vi "SetupEQE_ActiveX.vi"(6 "Skip?":bool, 8 "error in (no error)":errorcluster) -> (0 "error out":errorcluster)   [LabVIEW 2011]
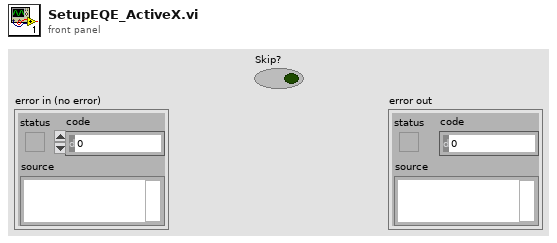
[diagram p1: front panel]
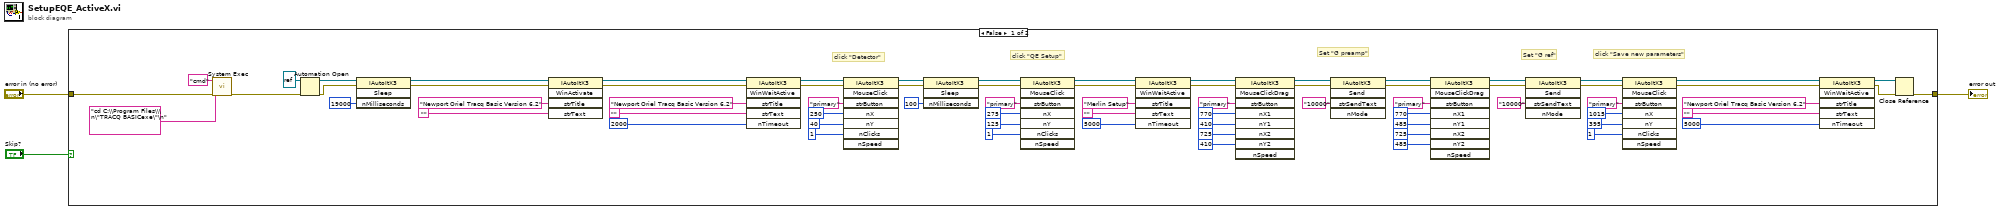
[diagram p0: block diagram]
diagram:
  n1 = case shown="False" "Skip?" {
    tunnel: "error in (no error)" -> [w6 w75]
    tunnel: [w72 w75] -> w2
    frame False {
      # "click \"Save new parameters\""
      # "Set \"G ref\""
      # "Set \"G preamp\""
      # "click \"QE Setup\""
      # "click \"Detector\""
      n2 = call <vilib>:"System Exec.vi"("error in (no error)"=w6, "standard input"="cd C:\\Program Files\\\n\"TRACQ BASICexe\"\n", "command line"="cmd") -> ("error out"=w5:errorcluster)  [unwired: 5 in, 3 out]
      n3 = Automation Open(error in (no error)=w5, Automation Refnum=refnum<k7> refnum ("AutoItX3Lib.IAutoItX3")) -> (Automation Refnum=w9:refnum<k7>, error out=w8:errorcluster)  [unwired: 2 in]
      n4 = invoke class="IAutoItX3" method="Sleep"(reference=w9, error in=w8, "nMilliseconds"=19000) -> (reference out=w70:refnum<k7>, error out=w71:errorcluster)  [unwired: 1 in, 2 out]
      n5 = invoke class="IAutoItX3" method="WinActivate"(reference=w70, error in=w71, "strTitle"="Newport Oriel Tracq Basic Version 6.2", "strText"="") -> (reference out=w69:refnum<k7>, error out=w62:errorcluster)  [unwired: 1 in, 3 out]
      n6 = invoke class="IAutoItX3" method="WinWaitActive"(reference=w69, error in=w62, "strTitle"="Newport Oriel Tracq Basic Version 6.2", "strText"="", "nTimeout"=2000) -> (reference out=w63:refnum<k7>, error out=w61:errorcluster)  [unwired: 1 in, 4 out]
      n7 = invoke class="IAutoItX3" method="MouseClick"(reference=w63, error in=w61, "strButton"="primary", "nX"=250, "nY"=40, "nClicks"=1) -> (reference out=w55:refnum<k7>, error out=w54:errorcluster)  [unwired: 2 in, 6 out]
      n8 = invoke class="IAutoItX3" method="Sleep"(reference=w55, error in=w54, "nMilliseconds"=100) -> (reference out=w49:refnum<k7>, error out=w48:errorcluster)  [unwired: 1 in, 2 out]
      n9 = invoke class="IAutoItX3" method="MouseClick"(reference=w49, error in=w48, "strButton"="primary", "nX"=275, "nY"=125, "nClicks"=1) -> (reference out=w44:refnum<k7>, error out=w43:errorcluster)  [unwired: 2 in, 6 out]
      n10 = invoke class="IAutoItX3" method="WinWaitActive"(reference=w44, error in=w43, "strTitle"="Merlin Setup", "strText"="", "nTimeout"=5000) -> (reference out=w42:refnum<k7>, error out=w41:errorcluster)  [unwired: 1 in, 4 out]
      n11 = invoke class="IAutoItX3" method="MouseClickDrag"(reference=w42, error in=w41, "strButton"="primary", "nX1"=770 ("nX"), "nY1"=410 ("nY"), "nX2"=725 ("nClicks"), "nY2"=410 ("nClicks")) -> (reference out=w35:refnum<k7>, error out=w34:errorcluster)  [unwired: 2 in, 7 out]
      n12 = invoke class="IAutoItX3" method="Send"(reference=w35, error in=w34, "strSendText"="10000") -> (reference out=w24:refnum<k7>, error out=w23:errorcluster)  [unwired: 2 in, 3 out]
      n13 = invoke class="IAutoItX3" method="MouseClickDrag"(reference=w24, error in=w23, "strButton"="primary", "nX1"=770 ("nX"), "nY1"=485 ("nY"), "nX2"=725 ("nClicks"), "nY2"=485 ("nClicks")) -> (reference out=w27:refnum<k7>, error out=w26:errorcluster)  [unwired: 2 in, 7 out]
      n14 = invoke class="IAutoItX3" method="Send"(reference=w27, error in=w26, "strSendText"="10000") -> (reference out=w18:refnum<k7>, error out=w17:errorcluster)  [unwired: 2 in, 3 out]
      n15 = invoke class="IAutoItX3" method="MouseClick"(reference=w18, error in=w17, "strButton"="primary", "nX"=1015, "nY"=395, "nClicks"=1) -> (reference out=w13:refnum<k7>, error out=w12:errorcluster)  [unwired: 2 in, 6 out]
      n16 = invoke class="IAutoItX3" method="WinWaitActive"(reference=w13, error in=w12, "strTitle"="Newport Oriel Tracq Basic Version 6.2", "strText"="", "nTimeout"=5000) -> (reference out=w11:refnum<k7>, error out=w10:errorcluster)  [unwired: 1 in, 4 out]
      n17 = Close Reference(reference=w11, error in (no error)=w10) -> (error out=w72:errorcluster)
    }
    frame True {
    }
  }
  "error out" <- w2
